vi "TærningeKast.vi"() -> ()   [LabVIEW 2022 SP3]
panel:
  in  "Antal sider":i32(slide) scale=0.0..64.0
  out "XY Graph":cluster{"Y":dbl[], "Y":dbl[]}[](graph)
  out "Sum af slag":i32
  out "sum af procent":dbl
  out "Procent array":dbl[](array[numeric])
  out "Udfalds array":i32[](array[numeric])
  in  "Andtal kast":i32
  in  "Andtal tærninger":i32
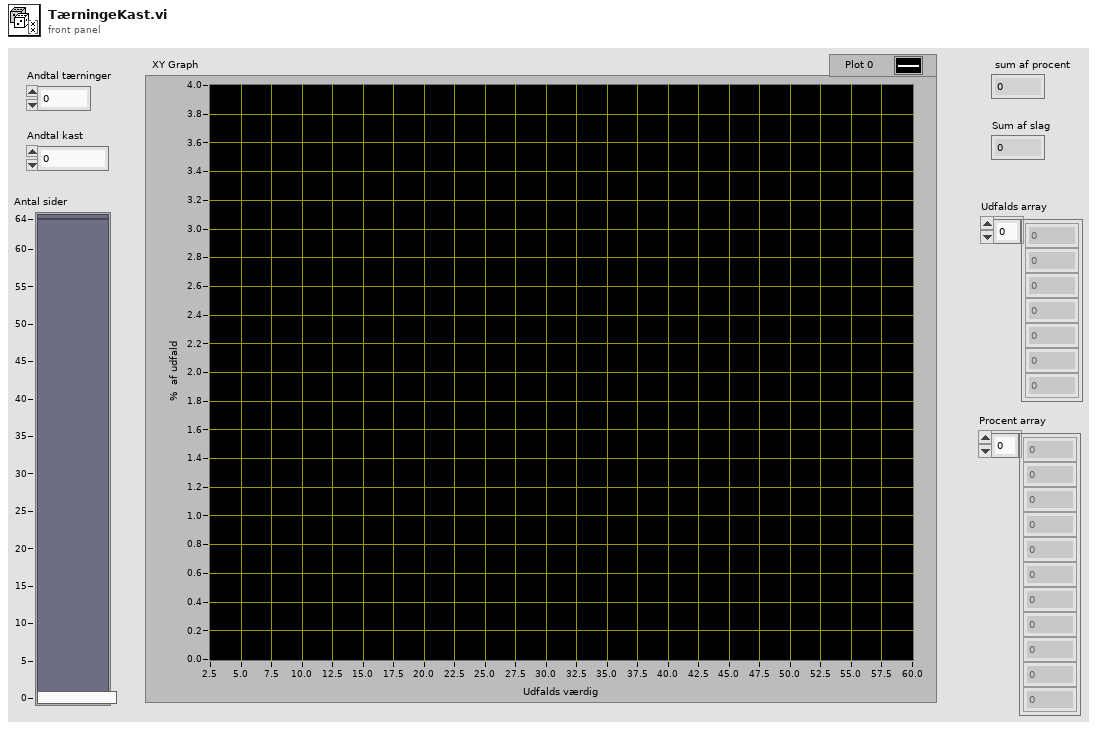
[diagram p1: front panel]
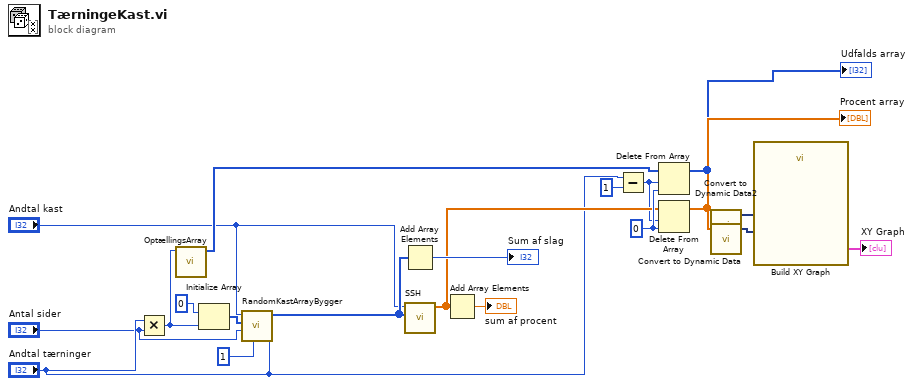
[diagram p0: block diagram]
diagram:
  w11 = 0 ("index")
  n1 = Multiply(x="Andtal tærninger", y="Antal sider") -> (x*y=w4:i32)
  n2 = call "OptællingsArray.vi"("Numeric"=w4) -> ("Array"=w10:i32[])  [unwired: 10 in]
  n3 = Initialize Array(0 ("element"), w4) -> (w12:i32[])
  n4 = call "RandomKastArrayBygger.vi"("Andtal tærninger"="Andtal tærninger", "Nedrre grænse"=1, "Øvre grænse"="Antal sider", "Array in"=w12, "Andtal kast"="Andtal kast") -> ("Array out"=w18:i32[])  [unwired: 6 in]
  n5 = Add Array Elements(numeric array=w18) -> (sum=→"Sum af slag":i32)
  n6 = call "SSH.vi"("Udkast array"=w18, "Andtal kast"="Andtal kast") -> ("Probabilitets array"=w9:dbl[])  [unwired: 9 in]
  n7 = Add Array Elements(numeric array=w9) -> (sum=→"sum af procent":dbl)
  n8 = Subtract(x="Andtal tærninger", y=1) -> (x-y=w8:i32)
  n9 = Delete From Array(array=w10, length=w8, index=w11) -> (array with subset deleted=w6:i32[])  [unwired: 1 out]
  "Udfalds array" <- w6
  n10 = Delete From Array(array=w9, length=w8, index=w11) -> (array with subset deleted=w7:dbl[])  [unwired: 1 out]
  "Procent array" <- w7
  n11 = call "Convert to Dynamic Data2"("Array"=w6) -> ("Dynamic Data Type"=w14:dynamicdata)  [unwired: 3 in]
  n12 = call "Convert to Dynamic Data"("Array"=w7) -> ("Dynamic Data Type"=w15:dynamicdata)  [unwired: 3 in]
  n13 = call "Build XY Graph"("Y Input"=w15, "X Input"=w14) -> ("XY Graph"=→"XY Graph":cluster{"X":dbl[], "Y":dbl[]}[])  [unwired: 8 in, 1 out]
